vi "Find Feature by Point.vi"(8 "error in":errorcluster, 11 "Point":T1) -> (0 "error out":errorcluster, 2 "Found?":bool, 3 "Feature":cluster{"name":string, "location":T1})   [LabVIEW 2019, in "route_guide_server.lvlib" / "RouteGuide.lvclass"]
uses:
  RouteGuide.lvclass
  RPC Messages/routeguide_Point.ctl
  route_guide_server.lvlib
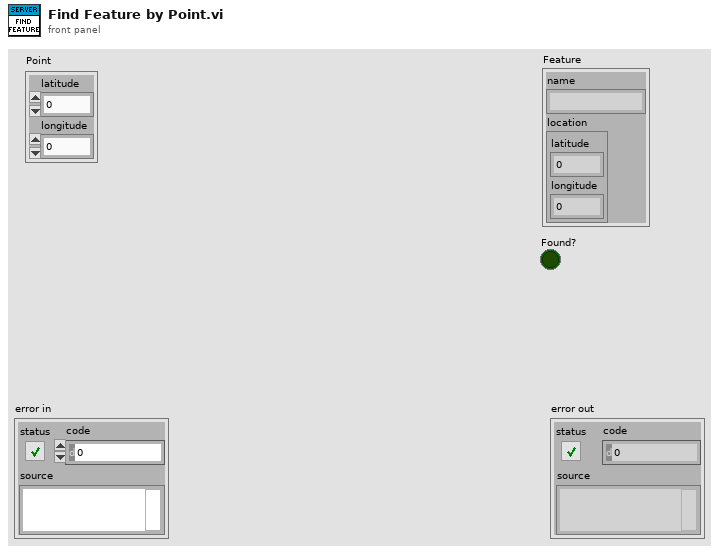
[diagram p1: front panel]
types:
  T1 = typedef "route_guide_server.lvlib/routeguide_Point.ctl" = cluster{"latitude":i32, "longitude":i32}
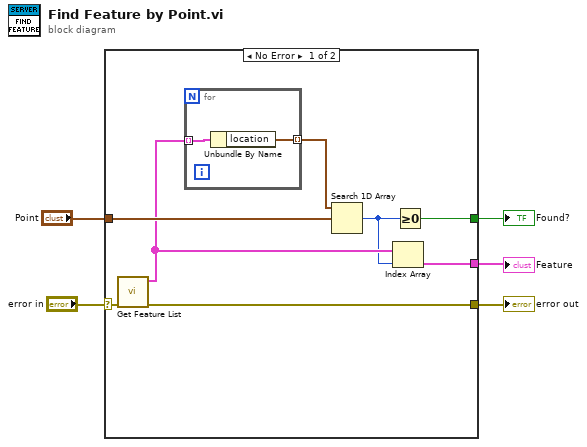
[diagram p0: block diagram]
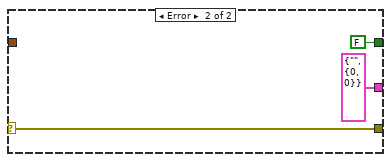
[diagram p2: hidden frame]
diagram:
  n1 = case shown="No Error" "error in" {
    selector: "error in" -> [w13 w18]
    tunnel: [w12 w18] -> w4
    tunnel: "Point" -> [w10 _]
    tunnel: [w7 cluster{"name":string, "location":T1} {"name"="", "location"={"latitude"=0, "longitude"=0}} ("routeguide_Feature")] -> w2
    tunnel: [w6 FALSE] -> w1
    frame No Error {
      n2 = call "Get Feature List.vi"("error in"=w13) -> ("error out"=w12:errorcluster, "Feature List"=w9:cluster{"name":string, "location":T1}[])  [unwired: 9 in]
      n3 = for {
        tunnel: w9 -> [w15] mode=indexing
        tunnel: [w14] -> w11 mode=indexing
        n4 = Unbundle By Name(w15) -> ("location"=w14:T1)
      }
      n5 = Search 1D Array(1D array=w11, element=w10) -> (index of element=w8:i32)  [unwired: 1 in]
      n6 = Index Array(array=w9, index=w8) -> (element=w7:cluster{"name":string, "location":T1})
      n7 = Greater Or Equal To 0?(x=w8) -> (x >= 0?=w6:bool)
    }
    frame Error {
    }
  }
  "error out" <- w4
  "Feature" <- w2
  "Found?" <- w1
